vi "ControlsPositionsStable.vi"(8 "error in (no error)":errorcluster, 11 "Referencia":T1) -> (0 "error out":errorcluster)   [LabVIEW 2021]
uses:
  Typedefs/Referencias.ctl
  Typedefs/Axis.ctl
  <vilib>/Utility/miscctls.llb/LVPointTypeDef.ctl
  <vilib>/Utility/miscctls.llb/LVRectTypeDef.ctl
  <vilib>/Utility/miscctls.llb/LVBoundsTypeDef.ctl
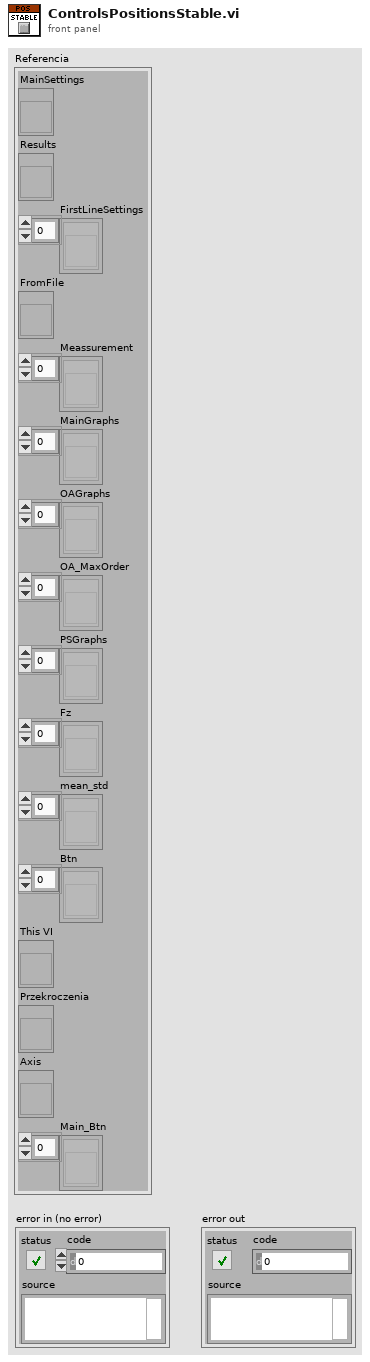
[diagram p1: front panel]
types:
  T1 = typedef "Referencias.ctl" = cluster{"MainSettings":refnum<vi>, "Results":refnum<vi>, "FirstLineSettings":refnum<vi>[], "FromFile":refnum<vi>, "Meassurement":refnum<vi>[], "MainGraphs":refnum<vi>[], "OAGraphs":refnum<vi>[], "OA_MaxOrder":refnum<vi>[], "PSGraphs":refnum<vi>[], "Fz":refnum<vi>[], "mean_std":refnum<vi>[], "Btn":refnum<vi>[], "This VI":refnum<vi>, "Przekroczenia":refnum<vi>, "Axis":refnum<vi>, "Main_Btn":refnum<vi>[]}
  T2 = enum32{"Invalid", "Standard", "Closed", "Hidden", "Minimized", "Maximized"}
  T3 = typedef "LVBoundsTypeDef.ctl" = cluster{"Width":u32, "Height":u32}
  T4 = typedef "LVRectTypeDef.ctl" = cluster{"Left":i16, "Top":i16, "Right":i16, "Bottom":i16}
  T5 = typedef "LVPointTypeDef.ctl" = cluster{"Horizontal":i16, "Vertical":i16}
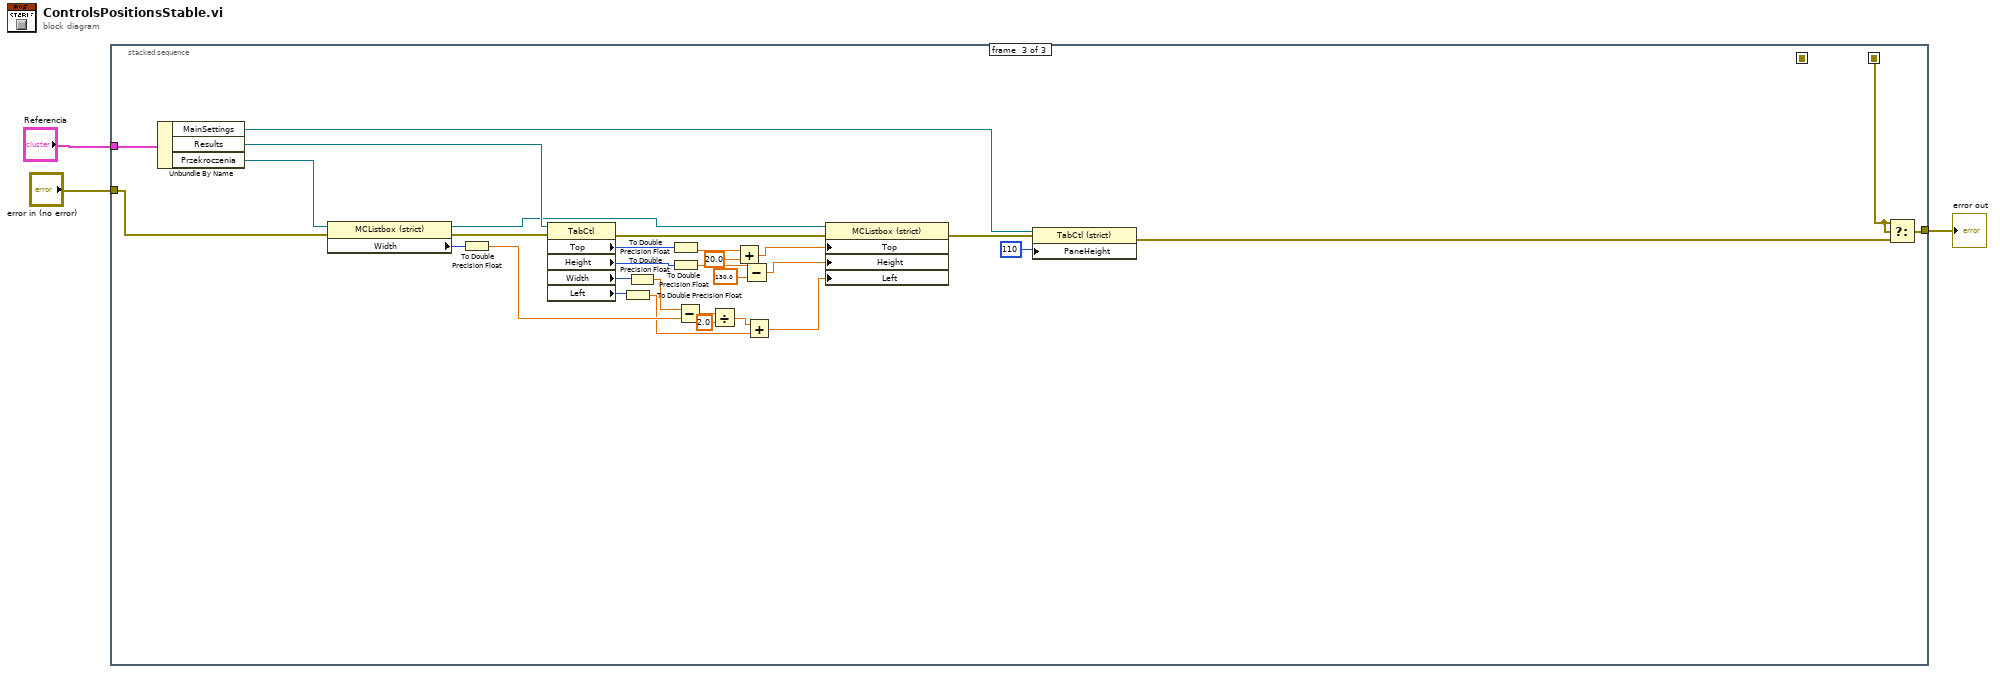
[diagram p0: block diagram]
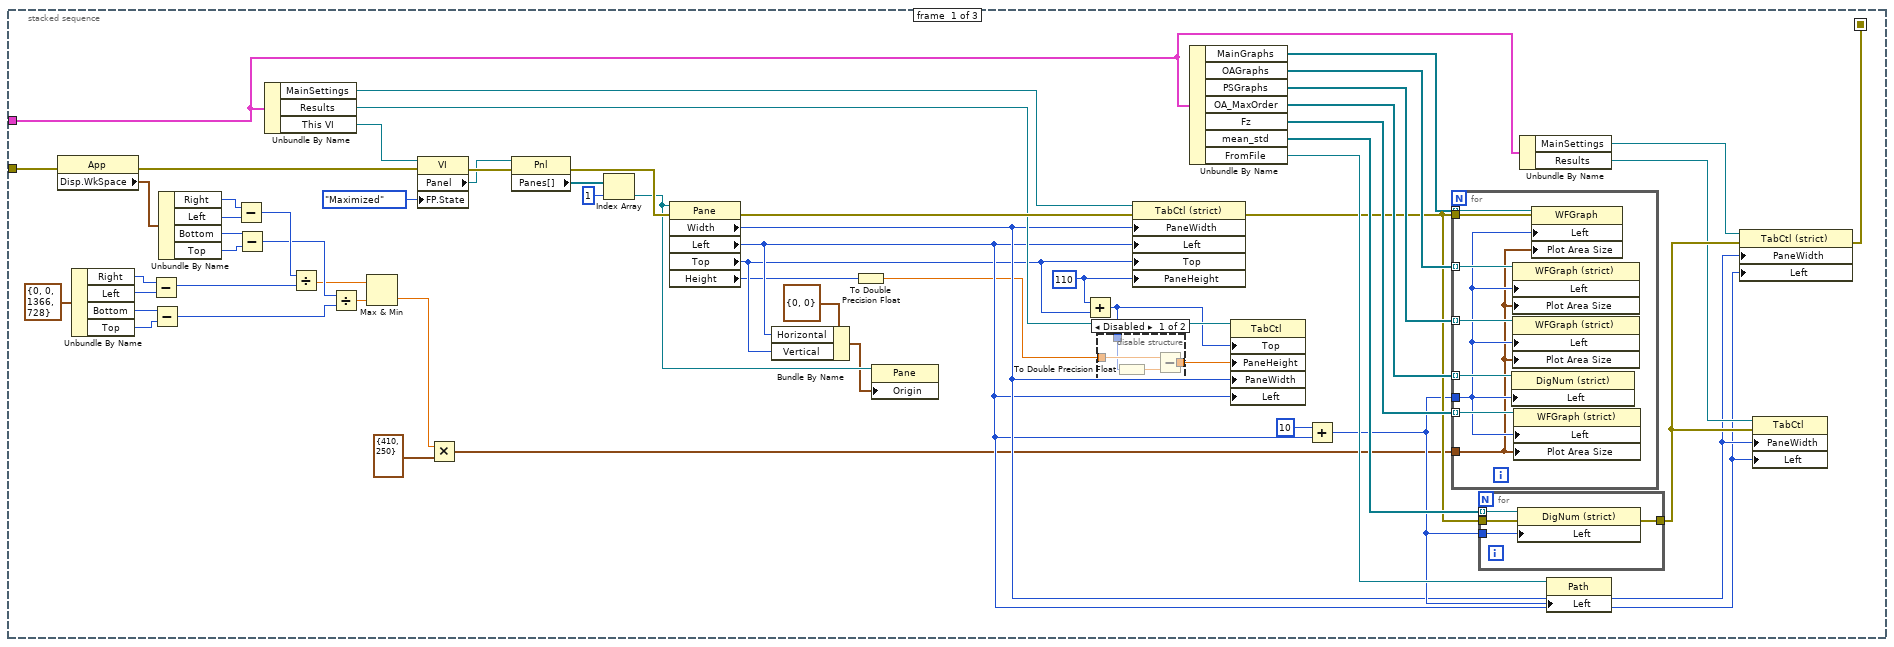
[diagram p2: hidden frame]
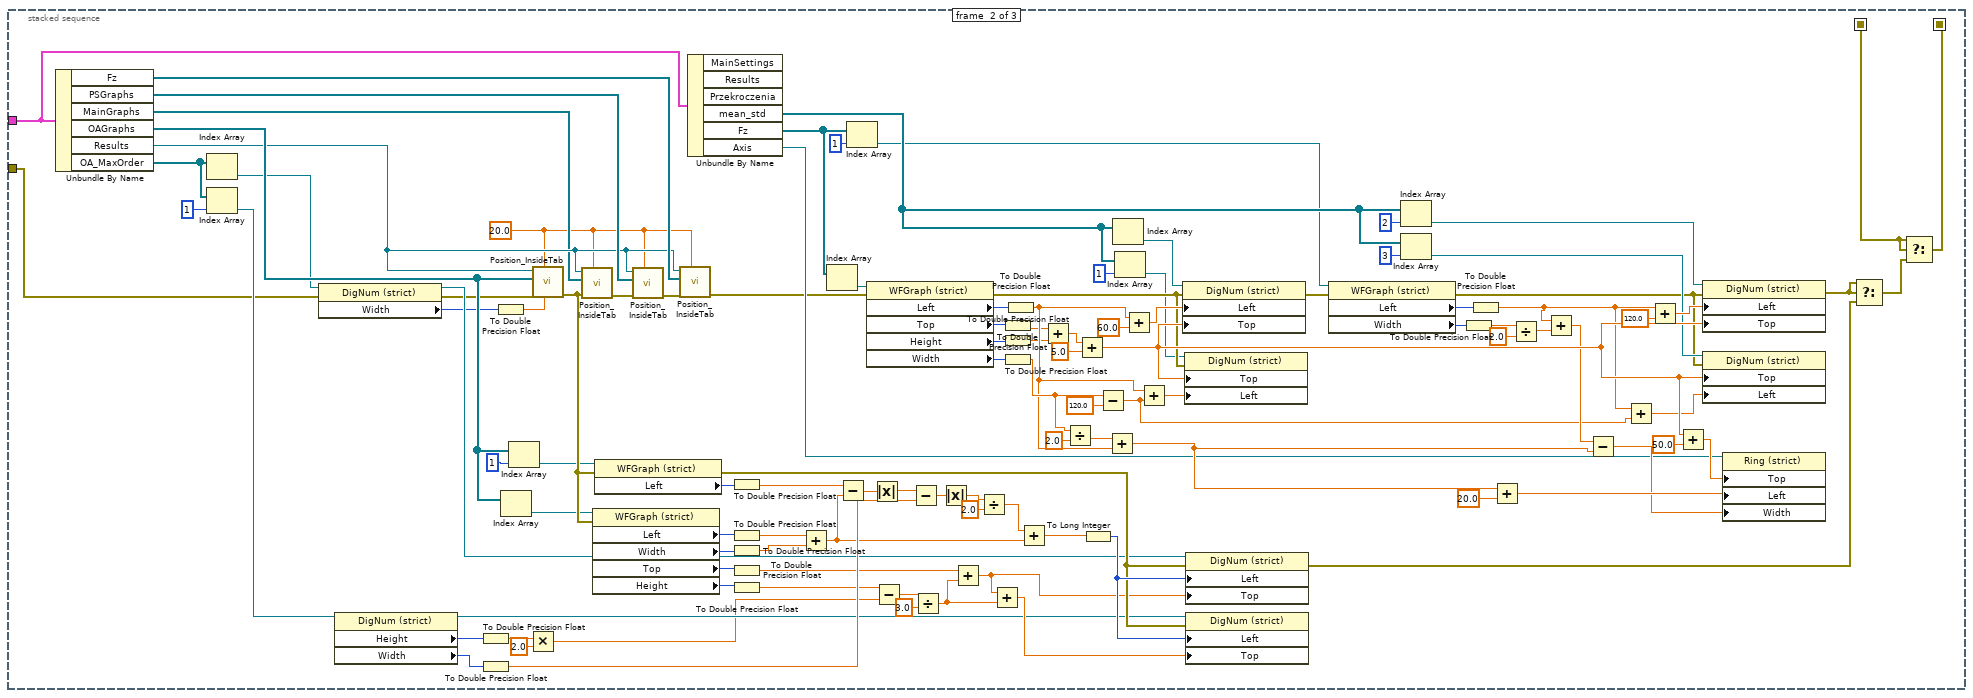
[diagram p4: hidden frame]
diagram:
  n1 = stacked-sequence {
    seq-local: [w4 _ _] -> [_ w80 _]
    seq-local: [_ w78 _] -> [_ _ w191]
    tunnel: "error in (no error)" -> [w36 w83 w192]
    tunnel: "Referencia" -> [w5 w84 w193]
    tunnel: [_ _ w189] -> w2
    frame #0 {
      w15 = u32 110 ("Tab Control Pane Dimension:Height")
      n2 = property class="App"(error in=w36) -> (error out=w35:errorcluster, "Disp.WkSpace"=w34:T4)  [unwired: 1 in, 1 out]
      n3 = Unbundle By Name(T4 {"Left"=0, "Top"=0, "Right"=1366, "Bottom"=728} ("Display:Primary Workspace")) -> ("Right"=w28:i16, "Left"=w27:i16, "Bottom"=w26:i16, "Top"=w25:i16)
      n4 = Subtract(x=w28, y=w27) -> (x-y=w23:i16)
      n5 = Subtract(x=w26, y=w25) -> (x-y=w21:i16)
      n6 = Unbundle By Name(w34) -> ("Right"=w33:i16, "Left"=w32:i16, "Bottom"=w31:i16, "Top"=w30:i16)
      n7 = Subtract(x=w33, y=w32) -> (x-y=w24:i16)
      n8 = Subtract(x=w31, y=w30) -> (x-y=w22:i16)
      n9 = Unbundle By Name(w5) -> ("MainSettings"=w55:refnum<vi>, "Results"=w54:refnum<vi>, "This VI"=w8:refnum<vi>)
      n10 = Divide(x=w24, y=w23) -> (x/y=w19:dbl)
      n11 = Divide(x=w22, y=w21) -> (x/y=w20:dbl)
      n12 = Max & Min(x=w19, y=w20) -> (min(x,y)=w18:dbl)  [unwired: 1 out]
      n13 = property class="VI"(reference=w8, error in=w35, "FP.State"=T2."Maximized" ("Front Panel Window:State")) -> (error out=w60:errorcluster, "Panel"=w59:refnum<vi>)  [unwired: 1 out]
      n14 = Multiply(x=w18, y=T3 {"Width"=410, "Height"=250} ("Plot Area Size")) -> (x*y=w16:cluster{"Width":dbl, "Height":dbl})
      n15 = property class="Pnl"(reference=w59, error in=w60) -> (error out=w56:errorcluster, "Panes[]"=w38:refnum<vi>[])  [unwired: 1 out]
      n16 = Index Array(array=w38, index=1) -> (element=w39:refnum<vi>)
      n17 = property class="Pane"(reference=w39, error in=w56) -> (error out=w58:errorcluster, "Width"=w42:u32, "Left"=w40:i32, "Top"=w14:i32, "Height"=w12:u32)  [unwired: 1 out]
      n18 = Bundle By Name(cluster=T5 {"Horizontal"=0, "Vertical"=0} ("Origin"), "Horizontal"=w40, "Vertical"=w14) -> (w37:T5)
      n19 = To Double Precision Float(number=w12) -> (double precision float=w11:dbl)
      n20 = property class="Pane"(reference=w39, "Origin"=w37) -> ()  [unwired: 1 in, 2 out]
      n21 = Add(x=w15, y=w14) -> (x+y=w10:u32)
      n22 = disable-structure shown="Disabled" {
        disable-tunnel: [w64 w65] -> w13
        disable-tunnel: w11 -> [w63 w65]
        disable-tunnel: w10 -> [w62 _]
        frame Disabled {
          n23 = To Double Precision Float(number=w62) -> (double precision float=w61:dbl)
          n24 = Subtract(x=w63, y=w61) -> (x-y=w64:dbl)
        }
        frame Enabled {
        }
      }
      n25 = property class="TabCtl (strict)"(reference=w55, error in=w58, "PaneWidth"=w42, "Left"=w40, "Top"=w14, "PaneHeight"=w15) -> (error out=w46:errorcluster)  [unwired: 1 out]
      n26 = Unbundle By Name(w5) -> ("MainGraphs"=w53:refnum<vi>[], "OAGraphs"=w52:refnum<vi>[], "PSGraphs"=w51:refnum<vi>[], "OA_MaxOrder"=w50:refnum<vi>[], "Fz"=w49:refnum<vi>[], "mean_std"=w47:refnum<vi>[], "FromFile"=w48:refnum<vi>)
      n27 = property class="TabCtl"(reference=w54, "Top"=w10, "PaneHeight"=w13, "PaneWidth"=w42, "Left"=w40) -> ()  [unwired: 1 in, 2 out]
      n28 = Add(x=10, y=w40) -> (x+y=w45:i32)
      n29 = for {
        tunnel: w45 -> [w71]
        tunnel: w53 -> [w77] mode=indexing
        tunnel: w52 -> [w76] mode=indexing
        tunnel: w51 -> [w75] mode=indexing
        tunnel: w50 -> [w74] mode=indexing
        tunnel: w46 -> [w73]
        tunnel: w49 -> [w72] mode=indexing
        tunnel: w16 -> [w70]
        n30 = property class="DigNum (strict)"(reference=w74, "Left"=w71) -> ()  [unwired: 1 in, 2 out]
        n31 = property class="WFGraph (strict)"(reference=w76, "Left"=w71, "Plot Area Size"=w70) -> ()  [unwired: 1 in, 2 out]
        n32 = property class="WFGraph (strict)"(reference=w75, "Left"=w71, "Plot Area Size"=w70) -> ()  [unwired: 1 in, 2 out]
        n33 = property class="WFGraph (strict)"(reference=w72, "Left"=w71, "Plot Area Size"=w70) -> ()  [unwired: 1 in, 2 out]
        n34 = property class="WFGraph"(reference=w77, error in=w73, "Left"=w71, "Plot Area Size"=w70) -> ()  [unwired: 2 out]
      }
      n35 = for {
        tunnel: w47 -> [w69] mode=indexing
        tunnel: w46 -> [w68]
        tunnel: w45 -> [w67]
        tunnel: [w66] -> w44
        n36 = property class="DigNum (strict)"(reference=w69, error in=w68, "Left"=w67) -> (error out=w66:errorcluster)  [unwired: 1 out]
      }
      n37 = Unbundle By Name(w5) -> ("MainSettings"=w6:refnum<vi>, "Results"=w43:refnum<vi>)
      n38 = property class="Path"(reference=w48, "Left"=w45) -> ()  [unwired: 1 in, 2 out]
      n39 = property class="TabCtl (strict)"(reference=w6, error in=w44, "PaneWidth"=w42, "Left"=w40) -> (error out=w4:errorcluster)  [unwired: 1 out]
      n40 = property class="TabCtl"(reference=w43, error in=w44, "PaneWidth"=w42, "Left"=w40) -> ()  [unwired: 2 out]
    }
    frame #1 {
      w86 = 20.0 ("Top")
      n41 = Unbundle By Name(w84) -> ("Fz"=w113:refnum<vi>[], "PSGraphs"=w112:refnum<vi>[], "MainGraphs"=w110:refnum<vi>[], "OAGraphs"=w114:refnum<vi>[], "Results"=w111:refnum<vi>, "OA_MaxOrder"=w108:refnum<vi>[])
      n42 = Index Array(array=w108) -> (element=w103:refnum<vi>)  [unwired: 1 in]
      n43 = Index Array(array=w108, index=1) -> (element=w115:refnum<vi>)
      n44 = property class="DigNum (strict)"(reference=w103, error in=w83) -> (reference out=w142:refnum<vi>, error out=w105:errorcluster, "Width"=w104:u32)
      n45 = property class="DigNum (strict)"(reference=w115) -> (reference out=w143:refnum<vi>, "Height"=w134:u32, "Width"=w135:u32)  [unwired: 1 in, 1 out]
      n46 = To Double Precision Float(number=w134) -> (double precision float=w133:dbl)
      n47 = To Double Precision Float(number=w135) -> (double precision float=w148:dbl)
      n48 = To Double Precision Float(number=w104) -> (double precision float=w109:dbl)
      n49 = Index Array(array=w114) -> (element=w116:refnum<vi>)  [unwired: 1 in]
      n50 = Index Array(array=w114, index=1) -> (element=w117:refnum<vi>)
      n51 = Multiply(x=w133, y=2.0) -> (x*y=w136:dbl)
      n52 = call "Position_InsideTab.vi"("Extra"=w109, "Top"=w86, "error in (no error)"=w105, "FirstLineSettings"=w114, "TabControl in"=w111) -> ("error out"=w123:errorcluster)  [unwired: 3 in, 3 out]
      n53 = call "Position_InsideTab.vi"("Top"=w86, "error in (no error)"=w123, "FirstLineSettings"=w110, "TabControl in"=w111) -> ("error out"=w106:errorcluster)  [unwired: 4 in, 3 out]
      n54 = property class="WFGraph (strict)"(reference=w116, error in=w123) -> ("Left"=w126:i32, "Width"=w127:u32, "Top"=w131:i32, "Height"=w132:u32)  [unwired: 2 out]
      n55 = property class="WFGraph (strict)"(reference=w117, error in=w123) -> (error out=w145:errorcluster, "Left"=w122:i32)  [unwired: 1 out]
      n56 = call "Position_InsideTab.vi"("Top"=w86, "error in (no error)"=w106, "FirstLineSettings"=w112, "TabControl in"=w111) -> ("error out"=w107:errorcluster)  [unwired: 4 in, 3 out]
      n57 = call "Position_InsideTab.vi"("Top"=w86, "error in (no error)"=w107, "FirstLineSettings"=w113, "TabControl in"=w111) -> ("error out"=w149:errorcluster)  [unwired: 4 in, 3 out]
      n58 = Unbundle By Name(w84) -> ("mean_std"=w165:refnum<vi>[], "Fz"=w150:refnum<vi>[], "Axis"=w174:refnum<vi>)  [unwired: 3 out]
      n59 = To Double Precision Float(number=w122) -> (double precision float=w118:dbl)
      n60 = To Double Precision Float(number=w126) -> (double precision float=w124:dbl)
      n61 = To Double Precision Float(number=w127) -> (double precision float=w125:dbl)
      n62 = To Double Precision Float(number=w131) -> (double precision float=w130:dbl)
      n63 = To Double Precision Float(number=w132) -> (double precision float=w128:dbl)
      n64 = Add(x=w124, y=w125) -> (x+y=w139:dbl)
      n65 = Index Array(array=w150) -> (element=w151:refnum<vi>)  [unwired: 1 in]
      n66 = Subtract(x=w118, y=w139) -> (x-y=w119:dbl)
      n67 = Index Array(array=w150, index=1) -> (element=w162:refnum<vi>)
      n68 = property class="WFGraph (strict)"(reference=w151, error in=w149) -> (error out=w159:errorcluster, "Left"=w170:i32, "Top"=w153:i32, "Height"=w154:u32, "Width"=w160:u32)  [unwired: 1 out]
      n69 = Absolute Value(x=w119) -> (abs(x)=w120:dbl)
      n70 = Subtract(x=w128, y=w136) -> (x-y=w129:dbl)
      n71 = Subtract(x=w120, y=w148) -> (x-y=w121:dbl)
      n72 = Divide(x=w129, y=3.0) -> (x/y=w140:dbl)
      n73 = Absolute Value(x=w121) -> (abs(x)=w138:dbl)
      n74 = Add(x=w130, y=w140) -> (x+y=w141:dbl)
      n75 = Divide(x=w138, y=2.0) -> (x/y=w137:dbl)
      n76 = Add(x=w141, y=w140) -> (x+y=w147:dbl)
      n77 = To Double Precision Float(number=w153) -> (double precision float=w156:dbl)
      n78 = To Double Precision Float(number=w154) -> (double precision float=w155:dbl)
      n79 = To Double Precision Float(number=w160) -> (double precision float=w185:dbl)
      n80 = To Double Precision Float(number=w170) -> (double precision float=w176:dbl)
      n81 = Add(x=w137, y=w139) -> (x+y=w144:dbl)
      n82 = Add(x=w156, y=w155) -> (x+y=w157:dbl)
      n83 = Divide(x=w185, y=2.0) -> (x/y=w175:dbl)
      n84 = Add(x=w157, y=5.0) -> (x+y=w183:dbl)
      n85 = To Long Integer(number=w144) -> (32bit integer=w146:i32)
      n86 = Subtract(x=w185, y=120.0) -> (x-y=w168:dbl)
      n87 = Add(x=w175, y=w176) -> (x+y=w186:dbl)
      n88 = Index Array(array=w165) -> (element=w152:refnum<vi>)  [unwired: 1 in]
      n89 = Index Array(array=w165, index=1) -> (element=w158:refnum<vi>)
      n90 = Add(x=w176, y=60.0) -> (x+y=w171:dbl)
      n91 = Add(x=w176, y=w168) -> (x+y=w167:dbl)
      n92 = property class="DigNum (strict)"(reference=w152, error in=w159, "Left"=w171, "Top"=w183) -> (error out=w161:errorcluster)  [unwired: 1 out]
      n93 = property class="DigNum (strict)"(reference=w158, error in=w159, "Top"=w183, "Left"=w167) -> ()  [unwired: 2 out]
      n94 = property class="DigNum (strict)"(reference=w142, error in=w145, "Left"=w146, "Top"=w141) -> (error out=w81:errorcluster)  [unwired: 1 out]
      n95 = property class="DigNum (strict)"(reference=w143, error in=w145, "Left"=w146, "Top"=w147) -> ()  [unwired: 2 out]
      n96 = property class="WFGraph (strict)"(reference=w162, error in=w161) -> (error out=w163:errorcluster, "Left"=w172:i32, "Width"=w177:u32)  [unwired: 1 out]
      n97 = Index Array(array=w165, index=2) -> (element=w164:refnum<vi>)
      n98 = Index Array(array=w165, index=3) -> (element=w166:refnum<vi>)
      n99 = To Double Precision Float(number=w177) -> (double precision float=w178:dbl)
      n100 = To Double Precision Float(number=w172) -> (double precision float=w180:dbl)
      n101 = Add(x=w186, y=20.0) -> (x+y=w187:dbl)
      n102 = Divide(x=w178, y=2.0) -> (x/y=w179:dbl)
      n103 = Add(x=w180, y=w179) -> (x+y=w181:dbl)
      n104 = Subtract(x=w181, y=w186) -> (x-y=w182:dbl)
      n105 = Add(x=w180, y=w168) -> (x+y=w169:dbl)
      n106 = Add(x=w180, y=120.0) -> (x+y=w173:dbl)
      n107 = Add(x=w183, y=50.0) -> (x+y=w184:dbl)
      n108 = property class="DigNum (strict)"(reference=w164, error in=w163, "Left"=w173, "Top"=w183) -> (error out=w82:errorcluster)  [unwired: 1 out]
      n109 = property class="DigNum (strict)"(reference=w166, error in=w163, "Top"=w183, "Left"=w169) -> ()  [unwired: 2 out]
      n110 = property class="Ring (strict)"(reference=w174, "Top"=w184, "Left"=w187, "Width"=w182) -> ()  [unwired: 1 in, 2 out]
      n111 = Select(t=w82, s=w82, f=w81) -> (s? t:f=w79:errorcluster)
      n112 = Select(t=w80, s=w80, f=w79) -> (s? t:f=w78:errorcluster)
    }
    frame #2 {
      n113 = Unbundle By Name(w193) -> ("MainSettings"=w216:refnum<vi>, "Results"=w217:refnum<vi>, "Przekroczenia"=w218:refnum<vi>)
      n114 = property class="MCListbox (strict)"(reference=w218, error in=w192) -> (reference out=w198:refnum<vi>, error out=w199:errorcluster, "Width"=w208:u32)
      n115 = To Double Precision Float(number=w208) -> (double precision float=w209:dbl)
      n116 = property class="TabCtl"(reference=w217, error in=w199) -> (error out=w200:errorcluster, "Top"=w204:i32, "Height"=w202:u32, "Width"=w210:u32, "Left"=w213:i32)  [unwired: 1 out]
      n117 = To Double Precision Float(number=w213) -> (double precision float=w188:dbl)
      n118 = To Double Precision Float(number=w210) -> (double precision float=w211:dbl)
      n119 = To Double Precision Float(number=w204) -> (double precision float=w205:dbl)
      n120 = To Double Precision Float(number=w202) -> (double precision float=w203:dbl)
      n121 = Subtract(x=w211, y=w209) -> (x-y=w212:dbl)
      n122 = Divide(x=w212, y=2.0) -> (x/y=w214:dbl)
      n123 = Add(x=w205, y=20.0) -> (x+y=w206:dbl)
      n124 = Subtract(x=w203, y=130.0) -> (x-y=w207:dbl)
      n125 = Add(x=w214, y=w188) -> (x+y=w215:dbl)
      n126 = property class="MCListbox (strict)"(reference=w198, error in=w200, "Top"=w206, "Height"=w207, "Left"=w215) -> (error out=w201:errorcluster)  [unwired: 1 out]
      n127 = property class="TabCtl (strict)"(reference=w216, error in=w201, "PaneHeight"=u32 110 ("Tab Control Pane Dimension:Height")) -> (error out=w190:errorcluster)  [unwired: 1 out]
      n128 = Select(t=w191, s=w191, f=w190) -> (s? t:f=w189:errorcluster)
    }
  }
  "error out" <- w2
